vi "Get PID Parameters (new).vi"(0 "setpoint":dbl format="%.2f", 1 "process variable":dbl format="%.2f", 2 "controller output":dbl format="%.2f", 3 "gain scheduling input":dbl format="%.2f", 4 "gain scheduling":T1={"gain schedule"=[100.0], "PID parameters"=[{"Kc"=0.0, "Ti (min)"=0.0, "Td (min)"=0.0}], "scheduling input"=0} {"scheduling input" items=["Setpoint", "Process variable", "Controller output", "Gain scheduling input"]; "PID parameters"."Td (min)" format="%.4f"; "PID parameters"."Ti (min)" format="%.4f"; "PID parameters"."Kc" format="%.4f"; "gain schedule" format="%.2f"}) -> (5 "PID parameters":cluster{"Kp":dbl, "Ti":dbl, "Td":dbl} {"Td" format="%.2f"; "Ti" format="%.2f"; "Kp" format="%.2f"}, 6 "scheduling index":i32)   [LabVIEW 2017, in "NI_PID__prctrl compat.lvlib"]
doc: "This VI selects the PID gains to be used from the gain schedule."
uses:
  <vilib>/addons/control/pid/NI_PID__prctrl compat.lvlib
panel:
  # "Get PID Parameters"
  # "Proportional gain or band (Kc)"
  # "Integral (reset) time (Ti, min)"
  # "Derivative (rate) time (Td, min)"
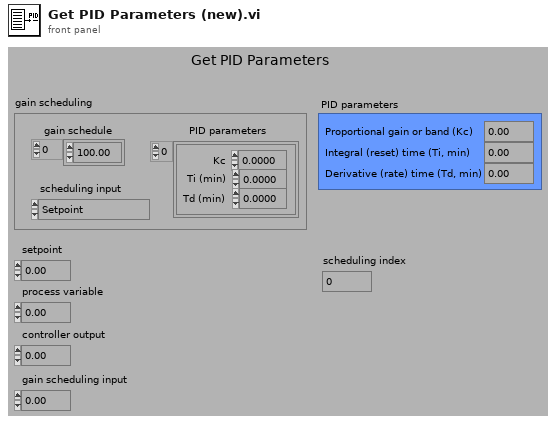
[diagram p1: front panel]
types:
  T1 = cluster{"gain schedule":dbl[], "PID parameters":cluster{"Kc":dbl, "Ti (min)":dbl, "Td (min)":dbl}[], "scheduling input":u16}
  T2 = cluster{"Kc":dbl, "Ti (min)":dbl, "Td (min)":dbl}[]
  T3 = cluster{"Kc":dbl, "Ti (min)":dbl, "Td (min)":dbl}
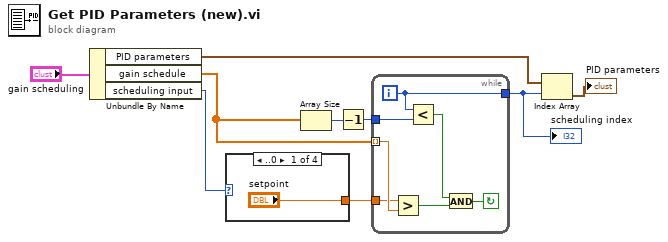
[diagram p0: block diagram]
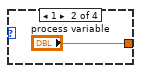
[diagram p2: hidden frame]
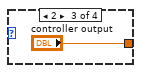
[diagram p3: hidden frame]
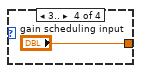
[diagram p4: hidden frame]
diagram:
  n1 = Unbundle By Name("gain scheduling") -> ("PID parameters"=w9:T2, "gain schedule"=w5:dbl[], "scheduling input"=w1:u16)
  n2 = case shown="..0" w1 {
    tunnel: ["setpoint" "process variable" "controller output" "gain scheduling input"] -> w2
    frame ..0 {
    }
    frame 1 {
    }
    frame 2 {
    }
    frame 3.. {
    }
  }
  n3 = Array Size(array=w5) -> (size(s)=w4:i32)
  n4 = Decrement(x=w4) -> (x-1=w3:i32)
  n5 = while {
    tunnel: w3 -> [w18]
    tunnel: w2 -> [w19]
    tunnel: [w17] -> w8
    tunnel: w5 -> [w20] mode=indexing
    i -> [w17]
    stop <- w14 continue-if-true
    n6 = Greater?(x=w19, y=w20) -> (0:w16:bool)
    n7 = Less?(x=w17, y=w18) -> (x < y?=w15:bool)
    n8 = And(x=w15, y=w16) -> (x .and. y?=w14:bool)
  }
  "scheduling index" <- w8
  n9 = Index Array(array=w9, index=w8) -> (element=→"PID parameters":T3)
